vi "Convert Detection Ball to AI Ball.vi"(7 "Lado":enum16{"Esquerdo", "Direito"}(ring) caption="Enum", 11 "Balls":refnum<class "Ball.lvclass">[](array[class])) -> (3 "Balls":refnum<class "Ball.lvclass">[](array[class]))   [LabVIEW 2018]
uses:
  Ball_class/Ball.lvclass
  Ball_class/Ball.lvclass/Ball.ctl
  Ball_class/Read Valid.vi
  Ball_class/Write v_x.vi
  Ball_class/Write v_y.vi
panel:
  out "Vel X":dbl
  out "Vel Y":dbl
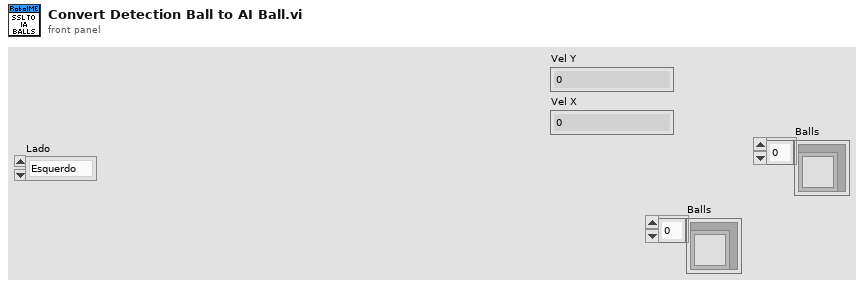
[diagram p1: front panel]
types:
  T1 = typedef "NI_Matrix.lvlib/RealMatrix.ctl" = dbl[][]
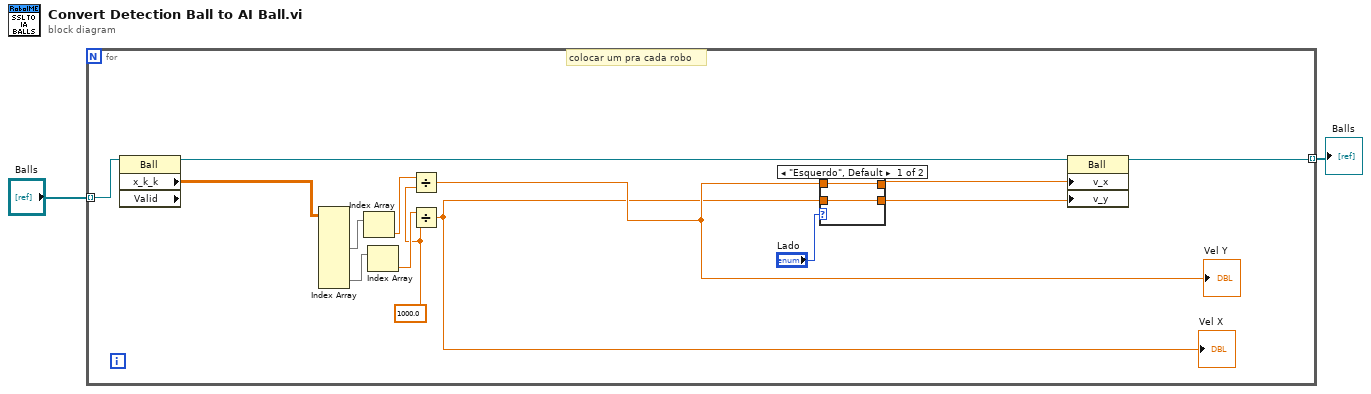
[diagram p0: block diagram]
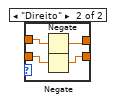
[diagram p2: hidden frame]
diagram:
  n1 = for {
    tunnel: "Balls" -> [w8] mode=indexing
    tunnel: [w3] -> w1 mode=indexing
    w12 = 1000.0
    # "colocar um pra cada robo"
    n2 = property class="Ball" props=["x_k_k", "Valid"](reference=w8) -> (reference out=w6:refnum<class "Ball.lvclass">, "x_k_k"=w7:T1)  [unwired: 1 in, 2 out]
    n3 = Index Array(array=w7) -> (element #2=w16:dbl[], element #4=w15:dbl[])  [unwired: 8 in, 2 out]
    n4 = Index Array(array=w16) -> (element=w14:dbl)  [unwired: 1 in]
    n5 = Index Array(array=w15) -> (element=w13:dbl)  [unwired: 1 in]
    n6 = Divide(x=w14, y=w12) -> (x/y=w10:dbl)
    "Vel Y" <- w10
    n7 = Divide(x=w13, y=w12) -> (x/y=w9:dbl)
    "Vel X" <- w9
    n8 = case shown="\"Esquerdo\", Default" "Lado" {
      tunnel: [w18 w22] -> w5
      tunnel: w10 -> [w18 w21]
      tunnel: [w17 w19] -> w4
      tunnel: w9 -> [w17 w20]
      frame "Esquerdo", Default {
      }
      frame "Direito" {
        n9 = Negate(x=w21) -> (-x=w22:dbl)
        n10 = Negate(x=w20) -> (-x=w19:dbl)
      }
    }
    n11 = property class="Ball"(reference=w6, "v_x"=w5, "v_y"=w4) -> (reference out=w3:refnum<class "Ball.lvclass">)  [unwired: 1 in, 1 out]
  }
  "Balls" <- w1
